vi "Cowl_Set.vi"   [LabVIEW 2019]
uses:
  Cowl_Globals.vi
  Cowl_States.ctl
types:
  T1 = typedef "Cowl_States.ctl" = enum16{"Manual_%VBus", "GoToAngle"}
  T2 = typedef "Cowl_Cluster.ctl" = cluster{"Control_State\n":T1, "Manual_Cowl_%Power":dbl}
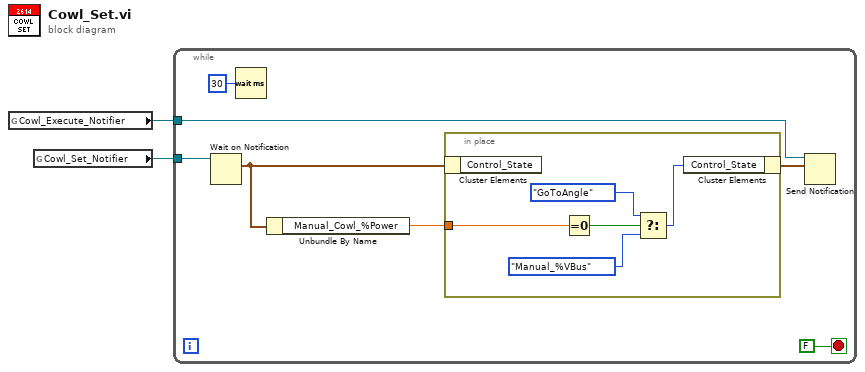
[diagram p0: block diagram]
diagram:
  n1 = global read "Cowl_Globals.vi" "Cowl_Execute_Notifier"() -> (w2:refnum<notifier>)
  n2 = global read "Cowl_Globals.vi" "Cowl_Set_Notifier"() -> (w1:refnum<notifier>)
  n3 = while {
    tunnel: w2 -> [w7]
    tunnel: w1 -> [w6]
    stop <- FALSE stop-if-true
    n4 = Wait on Notification(notifier=w6) -> (notification=w5:T2)  [unwired: 3 in, 3 out]
    n5 = Wait (ms)(milliseconds to wait=u32 30) -> ()  [unwired: 1 out]
    n6 = Unbundle By Name(w5) -> ("Manual_Cowl_%Power"=w4:dbl)
    n7 = in-place {
      in-place-border: w4 -> [w14]
      n8 = in-place-cluster #1(w5) -> ()  [unwired: 1 out]
      n9 = Equal To 0?(x=w14) -> (x = 0?=w12:bool)
      n10 = Select(t=Cowl_States."GoToAngle" ("Control_State"), s=w12, f=Cowl_States."Manual_%VBus" ("Control_State")) -> (s? t:f=w13:T1)
      n11 = in-place-cluster #1("Control_State"=w13) -> (w3:T2)
    }
    n12 = Send Notification(notification=w3, notifier=w7) -> ()  [unwired: 1 in, 2 out]
  }
